vi "test Add Find Remove RAF CD.vi"(8 "error in (no error)":errorcluster, 11 "TestCase in":refnum<class "Routing and Faulting Scripting Unit Tests.lvclass">) -> (0 "error out":errorcluster, 3 "TestCase out":refnum<class "Routing and Faulting Scripting Unit Tests.lvclass">)   [LabVIEW 2020, in "Routing and Faulting Scripting Unit Tests.lvclass"]
uses:
  Routing and Faulting Scripting Unit Tests.lvclass
  Routing and Faulting Scripting Unit Tests.lvclass/Routing and Faulting Scripting Unit Tests.ctl
  <vilib>/addons/_JKI Toolkits/VI Tester/TestCase.llb/TestCase.lvclass
  Routing and Faulting Scripting.lvlib
  C:/Program Files (x86)/National Instruments/LabVIEW 2020/vi.lib/addons/_JKI Toolkits/VI Tester/TestCase.llb/TestCase.lvclass
panel:
  in  "Save?":bool
  out "Output Filename":string
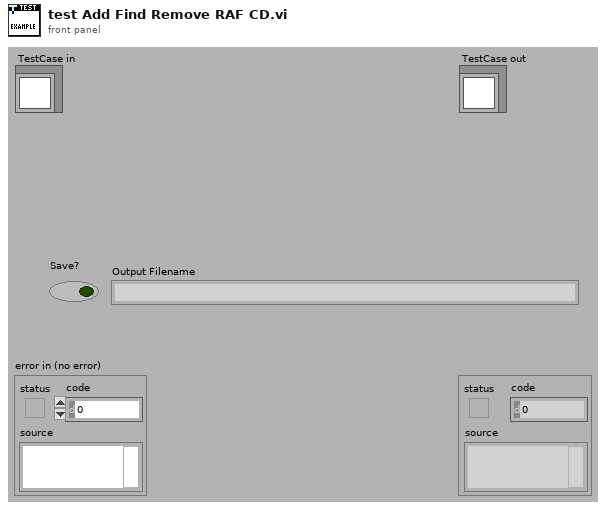
[diagram p1: front panel]
types:
  T1 = typedef "Custom Device API.lvlib/Custom Device Item Ref.ctl" = u64
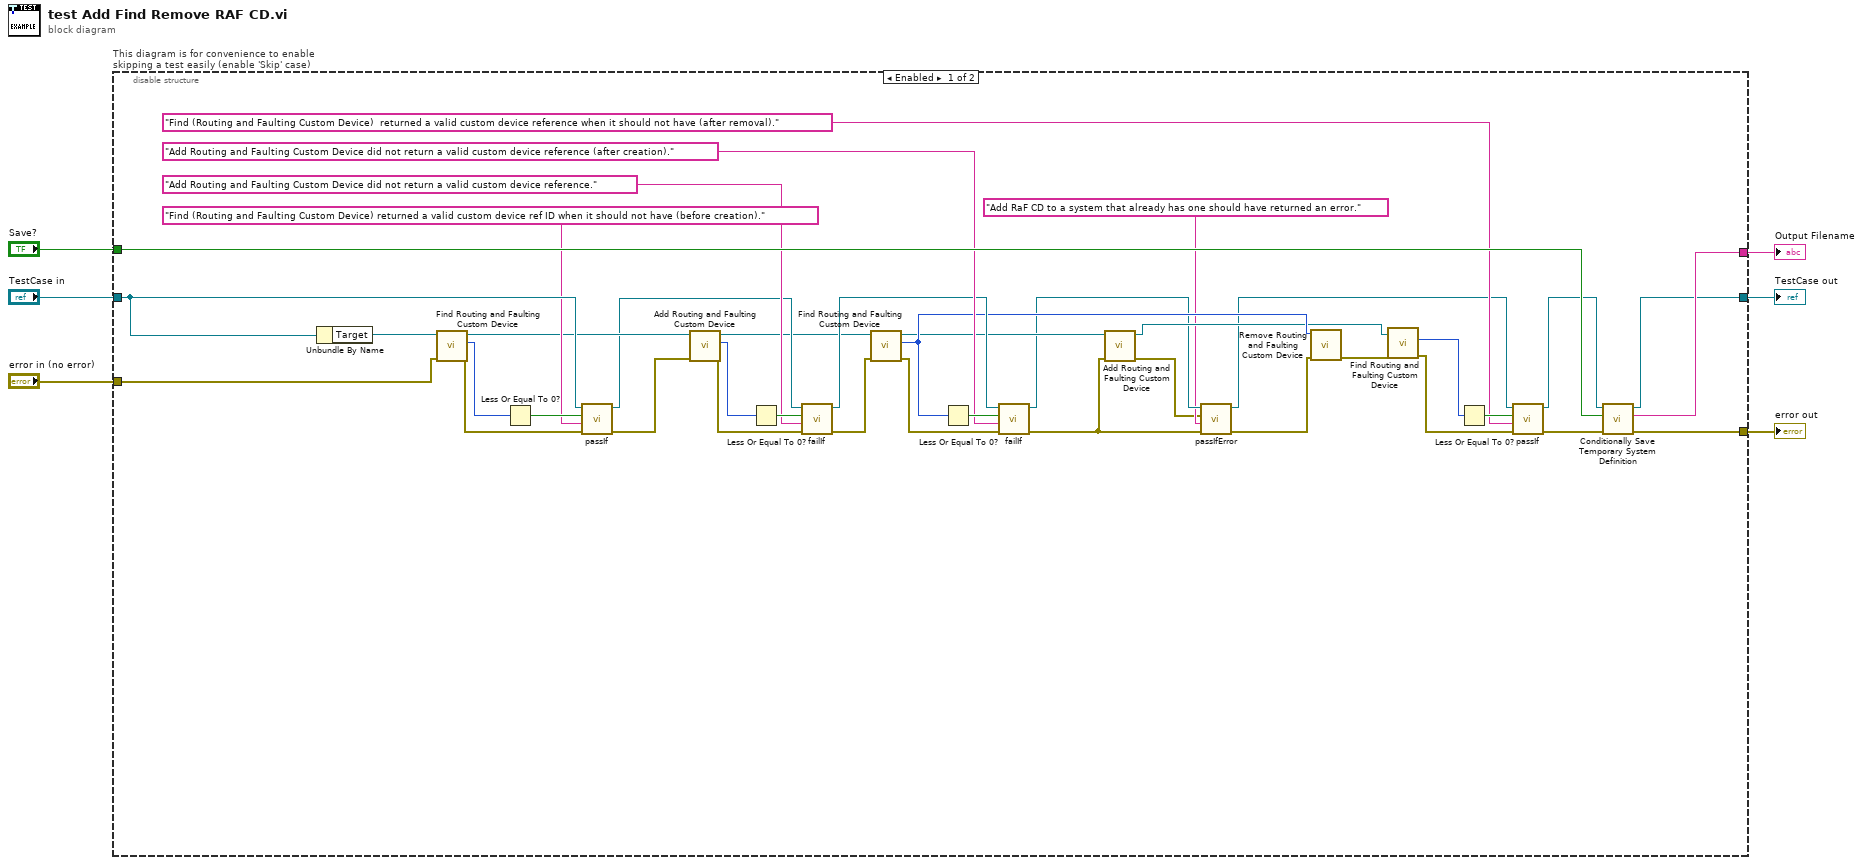
[diagram p0: block diagram]
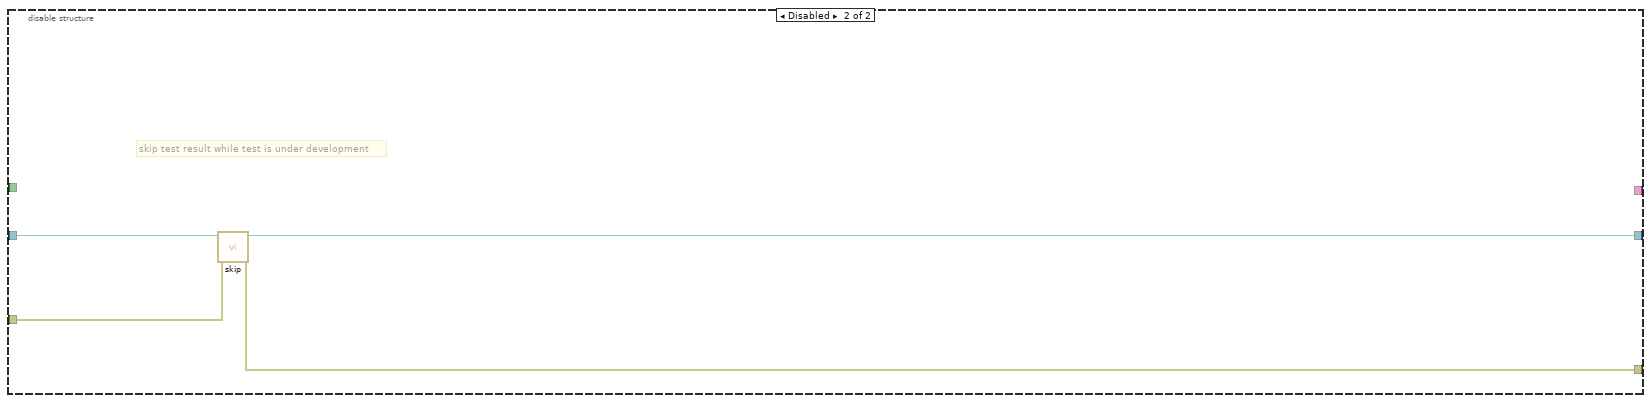
[diagram p2: hidden frame]
diagram:
  n1 = disable-structure "This diagram is for convenience to enable skipping a test easily (enable 'Skip' case)" shown="Enabled" {
    disable-tunnel: "TestCase in" -> [w40 w50]
    disable-tunnel: [w44 w48] -> w3
    disable-tunnel: [w45 w49] -> w5
    disable-tunnel: "error in (no error)" -> [w39 w47]
    disable-tunnel: [w46 _] -> w2
    disable-tunnel: "Save?" -> [w37 _]
    frame Enabled {
      n2 = Unbundle By Name(w40) -> ("Target"=w43:refnum<k24>)
      n3 = call "Find Routing and Faulting Custom Device.vi"("error in"=w39, "target in"=w43) -> ("error out"=w38:errorcluster, "routing and faulting custom device"=w42:T1, "target out"=w35:refnum<k24>)  [unwired: 7 in]
      n4 = Less Or Equal To 0?(x=w42) -> (x <= 0?=w41:bool)
      n5 = call-dynamic "passIf.vi"("error in (no error)"=w38, "message (\"\")"="Find (Routing and Faulting Custom Device) returned a valid custom device ref ID when it should not have (before creation)." ("message (\"\")"), "pass"=w41, "TestCase in"=w40) -> ("error out"=w34:errorcluster, "TestCase out"=w14:refnum<class "Routing and Faulting Scripting Unit Tests.lvclass">)  [unwired: 6 in]
      n6 = call "Add Routing and Faulting Custom Device.vi"("error in"=w34, "target in"=w35) -> ("error out"=w13:errorcluster, "routing and faulting custom device"=w33:T1, "target out"=w11:refnum<k24>)  [unwired: 7 in]
      n7 = Less Or Equal To 0?(x=w33) -> (x <= 0?=w32:bool)
      n8 = call-dynamic "failIf.vi"("error in (no error)"=w13, "message (\"\")"="Add Routing and Faulting Custom Device did not return a valid custom device reference." ("message (\"\")"), "fail"=w32, "TestCase in"=w14) -> ("error out"=w7:errorcluster, "TestCase out"=w28:refnum<class "Routing and Faulting Scripting Unit Tests.lvclass">)  [unwired: 6 in]
      n9 = call "Find Routing and Faulting Custom Device.vi"("error in"=w7, "target in"=w11) -> ("error out"=w12:errorcluster, "routing and faulting custom device"=w27:T1, "target out"=w19:refnum<k24>)  [unwired: 7 in]
      n10 = Less Or Equal To 0?(x=w27) -> (x <= 0?=w30:bool)
      n11 = call-dynamic "failIf.vi"("error in (no error)"=w12, "message (\"\")"="Add Routing and Faulting Custom Device did not return a valid custom device reference (after creation)." ("message (\"\")"), "fail"=w30, "TestCase in"=w28) -> ("error out"=w9:errorcluster, "TestCase out"=w17:refnum<class "Routing and Faulting Scripting Unit Tests.lvclass">)  [unwired: 6 in]
      n12 = call "Add Routing and Faulting Custom Device.vi"("error in"=w9, "target in"=w19) -> ("error out"=w10:errorcluster, "target out"=w18:refnum<k24>)  [unwired: 7 in, 1 out]
      n13 = call-dynamic "passIfError.vi"("error in (no error)"=w9, "task (\"\")"="Add RaF CD to a system that already has one should have returned an error." ("message (\"\")"), "error"=w10, "TestCase in"=w17) -> ("error out"=w8:errorcluster, "TestCase out"=w16:refnum<class "Routing and Faulting Scripting Unit Tests.lvclass">)  [unwired: 6 in]
      n14 = call "Remove Routing and Faulting Custom Device.vi"("error in"=w8, "routing and faulting custom device"=w27) -> ("error out"=w26:errorcluster)  [unwired: 9 in]
      n15 = call "Find Routing and Faulting Custom Device.vi"("error in"=w26, "target in"=w18) -> ("error out"=w24:errorcluster, "routing and faulting custom device"=w22:T1)  [unwired: 7 in, 1 out]
      n16 = Less Or Equal To 0?(x=w22) -> (x <= 0?=w25:bool)
      n17 = call-dynamic "passIf.vi"("error in (no error)"=w24, "message (\"\")"="Find (Routing and Faulting Custom Device)  returned a valid custom device reference when it should not have (after removal)." ("message (\"\")"), "pass"=w25, "TestCase in"=w16) -> ("error out"=w20:errorcluster, "TestCase out"=w23:refnum<class "Routing and Faulting Scripting Unit Tests.lvclass">)  [unwired: 6 in]
      n18 = call "Conditionally Save Temporary System Definition.vi"("error in (no error)"=w20, "Save?"=w37, "Test Case"=w23) -> ("error out"=w45:errorcluster, "filename"=w46:string, "Test Case"=w44:refnum<class "Routing and Faulting Scripting Unit Tests.lvclass">)  [unwired: 6 in]
    }
    frame Disabled {
      # "skip test result while test is under development"
      n19 = call <vilib>:"skip.vi"("error in (no error)"=w47, "TestCase in"=w50) -> ("error out"=w49:errorcluster, "TestCase out"=w48:refnum<class "Routing and Faulting Scripting Unit Tests.lvclass">)  [unwired: 8 in]
    }
  }
  "error out" <- w5
  "TestCase out" <- w3
  "Output Filename" <- w2
